vi "核对用户名称和密码.vi"(0 "用户密码":string, 1 "Data":string[][](array[string]), 2 "index of element":i32) -> (3 "登陆次数":string, 4 "布尔":bool, 5 "登陆时间":string, 6 "用户权限":string)   [LabVIEW 2013]
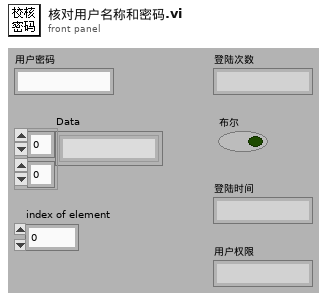
[diagram p1: front panel]
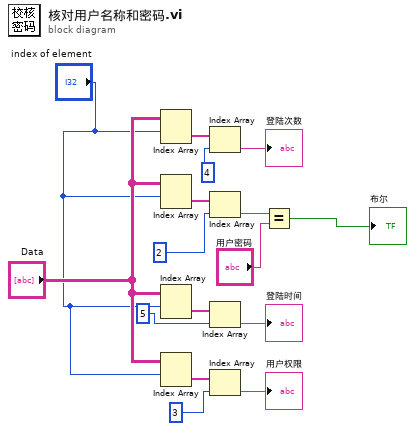
[diagram p0: block diagram]
diagram:
  n1 = Index Array(array="Data", index (row)="index of element") -> (element=w9:string[])  [unwired: 1 in]
  n2 = Index Array(array="Data", index (row)="index of element") -> (element=w6:string[])  [unwired: 1 in]
  n3 = Index Array(array="Data", index (row)="index of element") -> (element=w10:string[])  [unwired: 1 in]
  n4 = Index Array(array="Data", index (row)="index of element") -> (element=w11:string[])  [unwired: 1 in]
  n5 = Index Array(array=w9, index=4 ("索引")) -> (element=→"登陆次数":string)
  n6 = Index Array(array=w6, index=2 ("索引")) -> (element=w8:string)
  n7 = Index Array(array=w10, index=5 ("索引")) -> (element=→"登陆时间":string)
  n8 = Index Array(array=w11, index=3 ("索引")) -> (element=→"用户权限":string)
  n9 = Equal?(x=w8, y="用户密码") -> (x = y?=→"布尔":bool)
